vi "assemblies to tables.vi"(11 "assemblies":T1[](array[typedef])) -> (3 "Item Names":string[][](array[string]))   [LabVIEW 2013, in "EthernetIP editor node.lvclass"]
uses:
  EthernetIP editor node.lvclass
  <vilib>/NI/TBM Modules/Ethernet IP/configuration/assembly definition.ctl
  <vilib>/NI/TBM Modules/Ethernet IP/configuration/assembly type.ctl
  <vilib>/NI/TBM Modules/Ethernet IP/configuration/EthernetIP configuration.lvclass
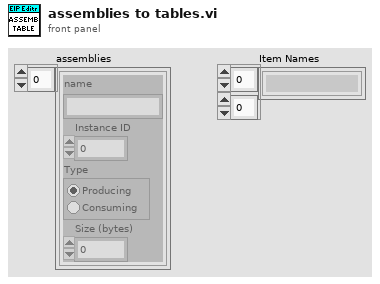
[diagram p1: front panel]
types:
  T1 = typedef "EthernetIP configuration.lvclass/assembly definition.ctl" = cluster{"name":string, "Instance ID":u32, "Type":T2, "Size (bytes)":u32}
  T2 = typedef "EthernetIP configuration.lvclass/assembly type.ctl" = enum32{"Producing", "Consuming"}
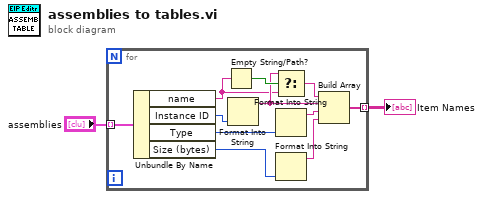
[diagram p0: block diagram]
diagram:
  n1 = for {
    tunnel: "assemblies" -> [w13] mode=indexing
    tunnel: [w7] -> w1 mode=indexing
    n2 = Unbundle By Name(w13) -> ("name"=w3:string, "Instance ID"=w10:u32, "Type"=w11:T2, "Size (bytes)"=w12:u32)
    n3 = Empty String/Path?(string/path=w3) -> (empty?=w6:bool)
    n4 = Format Into String(w10) -> (resulting string=w4:string)  [unwired: 3 in, 1 out]
    n5 = Select(t=w4, s=w6, f=w3) -> (s? t:f=w5:string)
    n6 = Format Into String(w11) -> (resulting string=w9:string)  [unwired: 3 in, 1 out]
    n7 = Format Into String(w12) -> (resulting string=w8:string)  [unwired: 3 in, 1 out]
    n8 = Build Array(w5, w4, w9, w8) -> (w7:string[])
  }
  "Item Names" <- w1
